vi "Concat 1D Variant Array.vi"(2 "error in (no error)":errorcluster, 3 "Array":variant[](array[variant])) -> (0 "error out":errorcluster, 1 "Variant":variant)   [LabVIEW 2020, in "LV Tiff.lvlib"]
uses:
  LV Tiff.lvlib
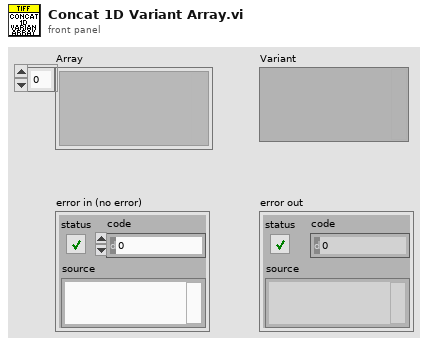
[diagram p1: front panel]
types:
  T1 = enum16{"big-endian, network order", "native, host order", "little-endian"}
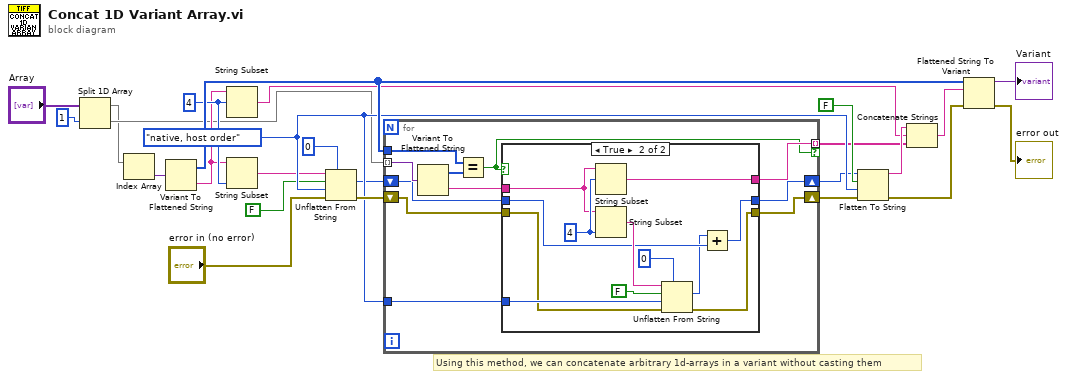
[diagram p0: block diagram]
diagram:
  w14 = 4 ("length (rest)")
  w18 = T1."native, host order" ("byte order (0:big-endian, network order)")
  # "Using this method, we can concatenate arbitrary 1d-arrays in a variant without casting them"
  n1 = Split 1D Array(array="Array", index=1) -> (first subarray=w7:variant[], second subarray=w9:variant[])
  n2 = Index Array(array=w7) -> (element=w8:variant)  [unwired: 1 in]
  n3 = Variant To Flattened String(Variant=w8) -> (data string=w12:string, 1:w20:i16[])
  n4 = String Subset(string=w12, offset (0)=w14) -> (substring=w2:string)  [unwired: 1 in]
  n5 = String Subset(string=w12, length (rest)=w14) -> (substring=w10:string)  [unwired: 1 in]
  n6 = Unflatten From String(type=0, binary string=w10, data includes array or string size? (T)=FALSE, byte order (0:big-endian, network order)=w18, error in (no error)="error in (no error)") -> (value=w15:i32, error out=w21:errorcluster)  [unwired: 1 out]
  n7 = for {
    tunnel: w18 -> [w32]
    tunnel: w9 -> [w36] mode=indexing
    shift-right: [w31] -> w16
    shift-left: w15 -> [w30]
    tunnel: w20 -> [w34]
    shift-right: [w27] -> w5
    shift-left: w21 -> [w28]
    tunnel: [w29] -> w1 mode=indexing if=w26
    n8 = Variant To Flattened String(Variant=w36) -> (data string=w35:string, 1:w33:i16[])
    n9 = Equal?(x=w34, y=w33) -> (x = y?=w26:bool)
    n10 = case shown="True" w26 {
      tunnel: w35 -> [_ w49]
      tunnel: w32 -> [_ w46]
      tunnel: [w38 w43] -> w31
      tunnel: w30 -> [w38 w44]
      tunnel: [_ w39] -> w29
      tunnel: w28 -> [w37 w41]
      tunnel: [w37 w40] -> w27
      frame False {
      }
      frame True {
        w50 = 4 ("length (rest)")
        n11 = String Subset(string=w49, offset (0)=w50) -> (substring=w39:string)  [unwired: 1 in]
        n12 = String Subset(string=w49, length (rest)=w50) -> (substring=w45:string)  [unwired: 1 in]
        n13 = Unflatten From String(type=0, binary string=w45, data includes array or string size? (T)=FALSE, byte order (0:big-endian, network order)=w46, error in (no error)=w41) -> (value=w42:i32, error out=w40:errorcluster)  [unwired: 1 out]
        n14 = Add(x=w42, y=w44) -> (x+y=w43:i32)
      }
    }
  }
  n15 = Flatten To String(anything=w16, prepend array or string size? (T)=FALSE, byte order (0:big-endian, network order)=w18, error in (no error)=w5) -> (data string=w3:string, error out=w4:errorcluster)  [unwired: 1 out]
  n16 = Concatenate Strings(w3, w2, w1) -> (w19:string)
  n17 = Flattened String To Variant(4:w4, 6:w19, 7:w20) -> (0:→"error out":errorcluster, 3:→"Variant":variant)
